vi "Single-Test-Case.vi"(11 "Power On?":bool) -> (3 "Test Case Passed":bool)   [LabVIEW 2018]
uses:
  Libraries/Device Under Test_Cloneable_DQMH/Device Under Test_Cloneable_DQMH.lvlib
panel:
  in  "Self Test Button":bool
  in  "Power Off Button":bool
  in  "Power On Button":bool
  # "This VI contains the test logic of the test cases."
  # "These buttons are not intended to be inputs. Their only goal is \nto be referenced internally by this VI."
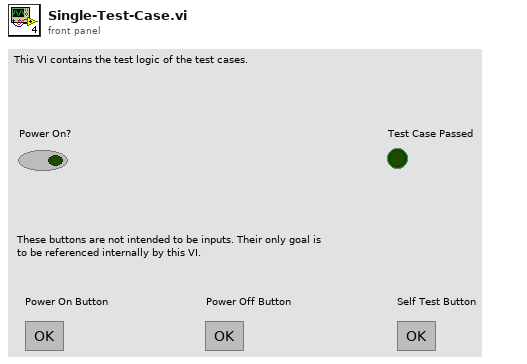
[diagram p1: front panel]
types:
  T1 = enum8{"Enabled", "Disabled", "Disabled and Grayed Out"}
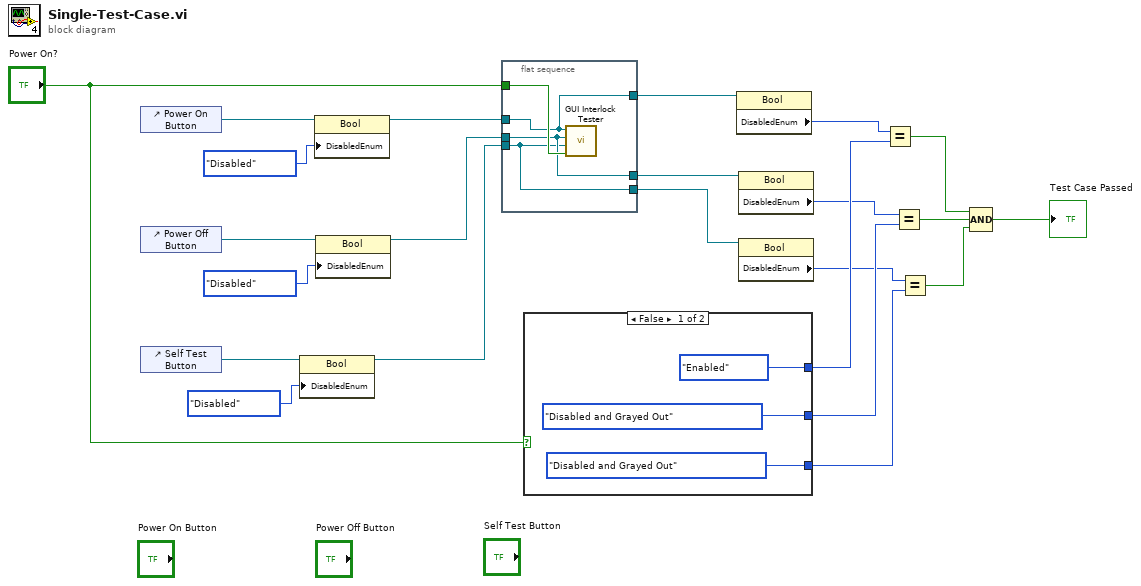
[diagram p0: block diagram]
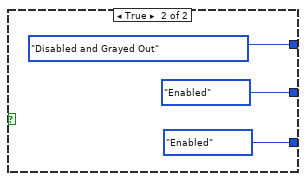
[diagram p2: hidden frame]
diagram:
  n1 = control-ref of="Power On Button"() -> (w23:refnum<vi>)
  n2 = control-ref of="Power Off Button"() -> (w19:refnum<vi>)
  n3 = control-ref of="Self Test Button"() -> (w18:refnum<vi>)
  n4 = property class="Bool"(reference=w18, "DisabledEnum"=T1."Disabled" ("Disabled")) -> (reference out=w15:refnum<vi>)  [unwired: 1 in, 1 out]
  n5 = property class="Bool"(reference=w23, "DisabledEnum"=T1."Disabled" ("Disabled")) -> (reference out=w17:refnum<vi>)  [unwired: 1 in, 1 out]
  n6 = property class="Bool"(reference=w19, "DisabledEnum"=T1."Disabled" ("Disabled")) -> (reference out=w16:refnum<vi>)  [unwired: 1 in, 1 out]
  n7 = flat-sequence {
    tunnel: w17 -> [w26]
    tunnel: w16 -> [w25]
    tunnel: w15 -> [w24]
    tunnel: "Power On?" -> [w27]
    tunnel: [w26] -> w14
    tunnel: [w25] -> w13
    tunnel: [w24] -> w12
    frame #0 {
      n8 = call "GUI Interlock Tester.vi"("Power State"=w27, "Self Test Button"=w24, "Power Off Button"=w25, "Power On Button"=w26) -> ()  [unwired: 8 in]
    }
  }
  n9 = case shown="False" "Power On?" {
    tunnel: [T1."Enabled" ("Disabled") T1."Disabled and Grayed Out" ("Disabled")] -> w11
    tunnel: [T1."Disabled and Grayed Out" ("Disabled") T1."Enabled" ("Disabled")] -> w9
    tunnel: [T1."Disabled and Grayed Out" ("Disabled") T1."Enabled" ("Disabled")] -> w6
    frame False {
    }
    frame True {
    }
  }
  n10 = property class="Bool"(reference=w14) -> ("DisabledEnum"=w10:T1)  [unwired: 1 in, 2 out]
  n11 = property class="Bool"(reference=w13) -> ("DisabledEnum"=w8:T1)  [unwired: 1 in, 2 out]
  n12 = property class="Bool"(reference=w12) -> ("DisabledEnum"=w7:T1)  [unwired: 1 in, 2 out]
  n13 = Equal?(x=w10, y=w11) -> (x = y?=w4:bool)
  n14 = Equal?(x=w8, y=w9) -> (x = y?=w3:bool)
  n15 = Equal?(x=w7, y=w6) -> (x = y?=w2:bool)
  n16 = Compound Arithmetic op=AND(w4, w3, w2) -> (→"Test Case Passed":bool)
